vi "ResetDCM1212(Host).vi"(0 "error in":errorcluster, 1 "FPGA Interface In":refnum<k20>) -> (2 "error out":errorcluster, 3 "LOCKED":bool, 4 "FPGA Interface Out":refnum<k20>)   [LabVIEW 2018]
uses:
  <vilib>/userdefined/High Color/nirio_resource_hc.ctl
  <vilib>/Utility/error.llb/Error Cluster From Error Code.vi
  <vilib>/rvi/errors/niLvFpgaAdjustHostInterfaceError.vi
  <vilib>/FPGAPlugInAG/Dynamic/niLvFpga_Close_Dynamic.vi
  <vilib>/rvi/interface/nirviReadWriteControl/nirviReadWriteControl.xnode
  <vilib>/rvi/interface/nirviCloseFPGA/nirviCloseFPGA.xnode
  NiFpgaLv.dll
  <vilib>/rvi/interface/Simulation/niFpgaSimulationCallBeginRW.vi
panel:
  in  "DEBUG":bool
  in  "resource name":T1="RIO0" caption="RIO Device"
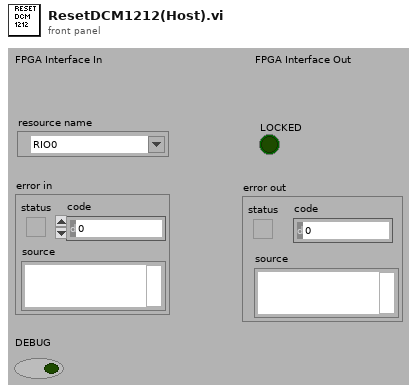
[diagram p1: front panel]
types:
  T1 = typedef "nirio_resource_hc.ctl" = tag
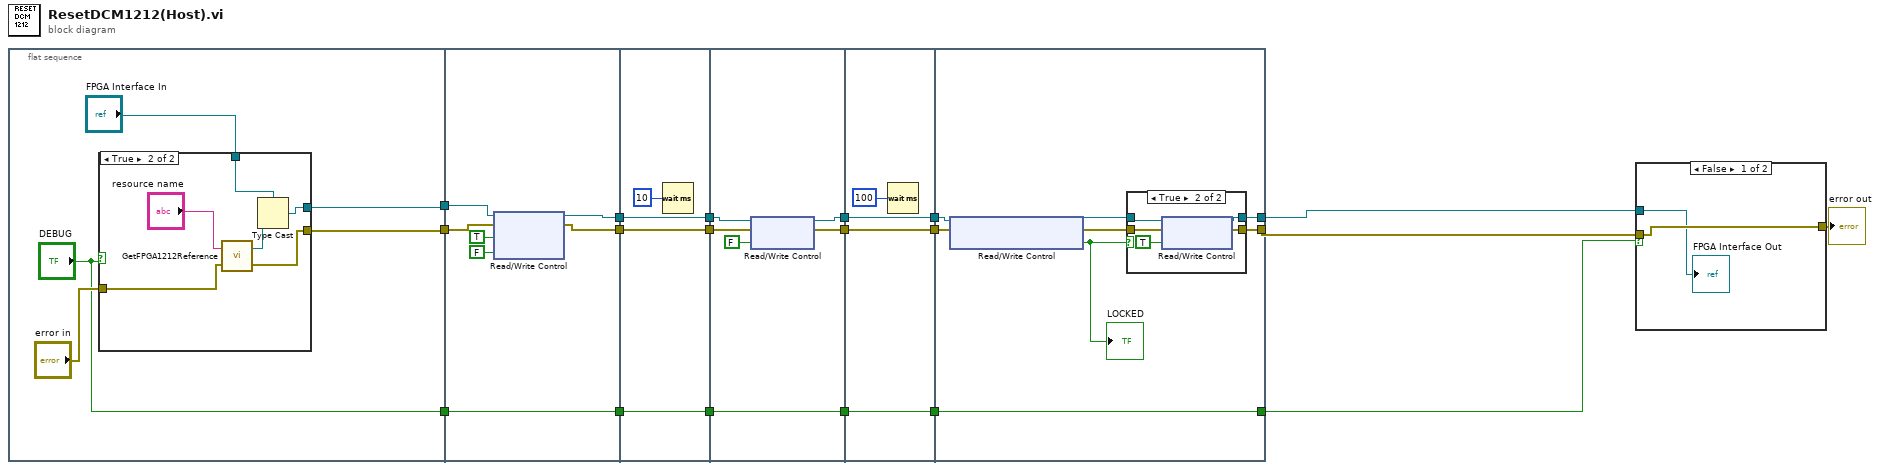
[diagram p0: block diagram]
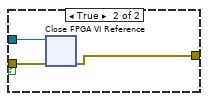
[diagram p2: hidden frame]
diagram:
  n1 = flat-sequence {
    tunnel: [w22] -> w9
    tunnel: [w21] -> w8
    tunnel: ["DEBUG"] -> w1
    tunnel: [w39] -> w17
    tunnel: [w37] -> w14
    tunnel: w9 -> [w36]
    tunnel: w8 -> [w38]
    tunnel: [w33] -> w2
    tunnel: w1 -> [w33]
    tunnel: [w42] -> w18
    tunnel: w17 -> [w42]
    tunnel: [w41] -> w15
    tunnel: w14 -> [w41]
    tunnel: [w40] -> w3
    tunnel: w2 -> [w40]
    tunnel: [w49] -> w19
    tunnel: w18 -> [w48]
    tunnel: w15 -> [w47]
    tunnel: [w46] -> w12
    tunnel: [w44] -> w4
    tunnel: w3 -> [w44]
    tunnel: w19 -> [w52]
    tunnel: [w52] -> w16
    tunnel: [w51] -> w13
    tunnel: w12 -> [w51]
    tunnel: [w50] -> w5
    tunnel: w4 -> [w50]
    tunnel: w16 -> [w61]
    tunnel: w13 -> [w60]
    tunnel: [w57] -> w11
    tunnel: [w56] -> w10
    tunnel: [w54] -> w6
    tunnel: w5 -> [w54]
    frame #0 {
      n2 = case shown="True" "DEBUG" {
        tunnel: [w25 w31] -> w22
        tunnel: [w26 w27] -> w21
        tunnel: "error in" -> [w26 w29]
        tunnel: "FPGA Interface In" -> [w25 w32]
        frame False {
        }
        frame True {
          n3 = call "GetFPGA1212Reference.vi"("error in"=w29, "RIO Device IN"="resource name") -> ("error out"=w27:errorcluster, "FPGA VI Reference Out"=w28:refnum<k20>)
          n4 = Type Cast(type=w32, x=w28) -> (*(type *) &x=w31:refnum<k20>)
        }
      }
    }
    frame #1 {
      n5 = xnode "Read/Write Control"("FPGA VI Reference In"=w36, "error in"=w38, "SysReset"=TRUE, "ClkEnable"=FALSE) -> ("FPGA VI Reference Out"=w39:refnum<k20>, "error out"=w37:errorcluster)
    }
    frame #2 {
      n6 = Wait (ms)(milliseconds to wait=u32 10) -> ()  [unwired: 1 out]
    }
    frame #3 {
      n7 = xnode "Read/Write Control"("FPGA VI Reference In"=w48, "error in"=w47, "SysReset"=FALSE ("WRITE MEM")) -> ("FPGA VI Reference Out"=w49:refnum<k20>, "error out"=w46:errorcluster)
    }
    frame #4 {
      n8 = Wait (ms)(milliseconds to wait=u32 100) -> ()  [unwired: 1 out]
    }
    frame #5 {
      n9 = xnode "Read/Write Control"("FPGA VI Reference In"=w61, "error in"=w60) -> ("FPGA VI Reference Out"=w59:refnum<k20>, "error out"=w58:errorcluster, "IO Module\\lockedfast"=w55:bool)
      "LOCKED" <- w55
      n10 = case shown="True" w55 {
        tunnel: w59 -> [w63 w68]
        tunnel: w58 -> [w62 w67]
        tunnel: [w62 w66] -> w57
        tunnel: [w63 w65] -> w56
        frame False {
        }
        frame True {
          n11 = xnode "Read/Write Control"("FPGA VI Reference In"=w68, "error in"=w67, "ClkEnable"=TRUE) -> ("FPGA VI Reference Out"=w65:refnum<k20>, "error out"=w66:errorcluster)
        }
      }
    }
  }
  n12 = case shown="False" w6 {
    tunnel: w11 -> [w70 w73]
    tunnel: w10 -> [w69 w72]
    tunnel: [w70 w71] -> w7
    frame False {
      "FPGA Interface Out" <- w69
    }
    frame True {
      n13 = xnode "Close FPGA VI Reference"("FPGA VI Reference In"=w72, "error in"=w73) -> ("error out"=w71:errorcluster)
    }
  }
  "error out" <- w7
